vi "Shutdown.vi"(8 "error in (no error)":errorcluster, 11 "Camera_Prime95B in":refnum<class "Camera_Prime95B.lvclass">) -> (0 "error out":errorcluster, 3 "Camera_Prime95B out":refnum<class "Camera_Prime95B.lvclass">)   [LabVIEW 2020, in "Camera_Prime95B.lvlib" / "Camera_Prime95B.lvclass"]
uses:
  Camera_Prime95B.lvclass
  Camera_Prime95B.lvclass/Camera_Prime95B.ctl
  E:/Development/DevHardSoftware/MMicroscopyAF/Model/Real Hardware/Camera_Prime95B/Camera_Prime95B/Dependencies/PVCamNET.dll
  Dependencies/PVCamNET.dll
  HAL Layer/Component/Camera/Camera/Camera.lvclass
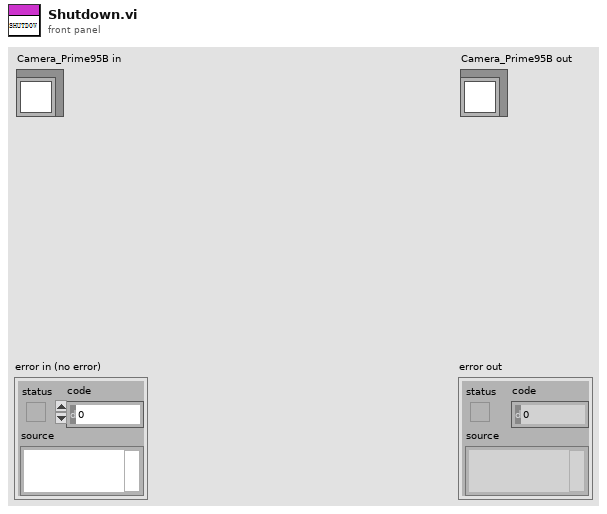
[diagram p1: front panel]
types:
  T1 = cluster{"Library Refnum":refnum<k24>, "Camera Refnum":refnum<k24>, "Status Callback Refnum":refnum<k27>, "New Frame Callback Refnum":refnum<k27>}
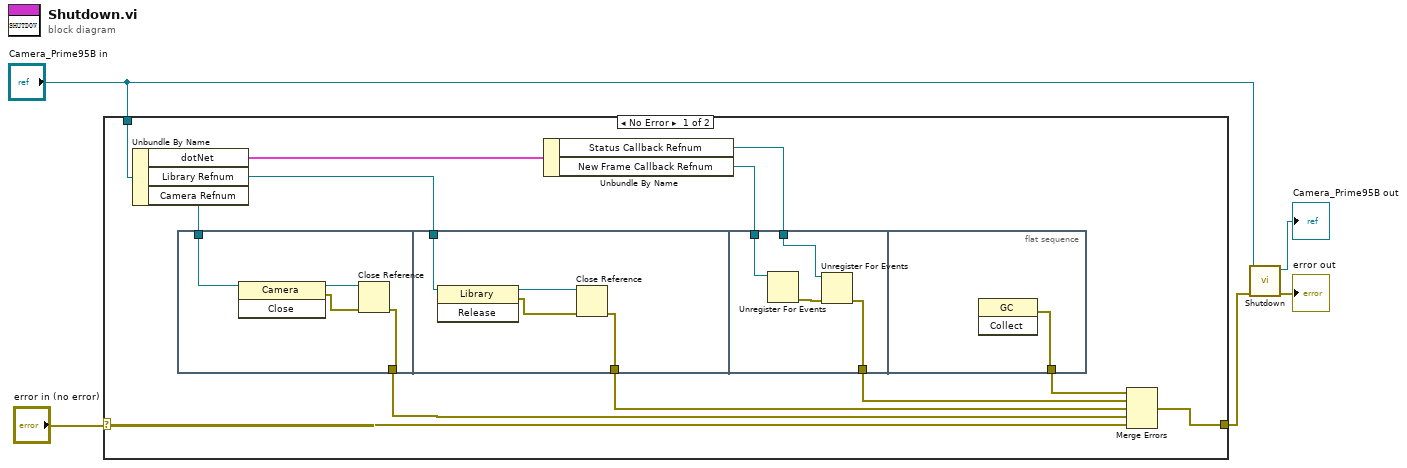
[diagram p0: block diagram]
diagram:
  n1 = case shown="No Error" "error in (no error)" {
    selector: "error in (no error)" -> [w11 w31]
    tunnel: [w10 w31] -> w2
    tunnel: "Camera_Prime95B in" -> [w17 _]
    frame No Error {
      n2 = Unbundle By Name(w17) -> ("dotNet"=w14:T1, "Library Refnum"=w15:refnum<k24>, "Camera Refnum"=w16:refnum<k24>)
      n3 = flat-sequence {
        tunnel: w16 -> [w21]
        tunnel: [w18] -> w9
        tunnel: w15 -> [w25]
        tunnel: [w22] -> w8
        tunnel: w13 -> [w27]
        tunnel: w12 -> [w28]
        tunnel: [w26] -> w7
        tunnel: [w30] -> w6
        frame #0 {
          n4 = invoke class="Camera" method="Close"(reference=w21) -> (reference out=w20:refnum<k24>, error out=w19:errorcluster)  [unwired: 2 in, 1 out]
          n5 = Close Reference(reference=w20, error in (no error)=w19) -> (error out=w18:errorcluster)
        }
        frame #1 {
          n6 = invoke class="Library" method="Release"(reference=w25) -> (reference out=w23:refnum<k24>, error out=w24:errorcluster)  [unwired: 2 in, 1 out]
          n7 = Close Reference(reference=w23, error in (no error)=w24) -> (error out=w22:errorcluster)
        }
        frame #2 {
          n8 = Unregister For Events(event registration refnum=w28) -> (error out=w29:errorcluster)  [unwired: 1 in]
          n9 = Unregister For Events(event registration refnum=w27, error in=w29) -> (error out=w26:errorcluster)
        }
        frame #3 {
          n10 = invoke class="GC" method="Collect"() -> (error out=w30:errorcluster)  [unwired: 3 in, 2 out]
        }
      }
      n11 = Unbundle By Name(w14) -> ("Status Callback Refnum"=w13:refnum<k27>, "New Frame Callback Refnum"=w12:refnum<k27>)
      n12 = Merge Errors(w6, w7, w8, w9, w11) -> (w10:errorcluster)
    }
    frame Error {
    }
  }
  n13 = call-parent "Shutdown.vi"("error in (no error)"=w2, "Camera in"="Camera_Prime95B in") -> ("error out"=→"error out":errorcluster, "Camera out"=→"Camera_Prime95B out":refnum<class "Camera_Prime95B.lvclass">)  [unwired: 8 in]
